vi "Trim All Quots String _APTLib.vi"(7 "Case (NoChange)":T1, 10 "location (both)":T2 items=["both", "start of string", "end of string"], 11 "String In":string) -> (3 "String Out":string)   [LabVIEW 2019]
doc: "This VI is Developed by Anish Prabu.\n\nCopyright © 2006, email:anishprabu243@yahoo.co.in.\nAll rights reserved."
uses:
  <userlib>/APTLib.lnk/String/_Trim String _APTLib.llb/WS _APTLib.ctl
  <userlib>/APTLib.lnk/String/_Trim String _APTLib.llb/Change Case Selector _APTLib.ctl
  <userlib>/APTLib.lnk/String/_Trim String _APTLib.llb/Trim WS (String) _APTLib.vi
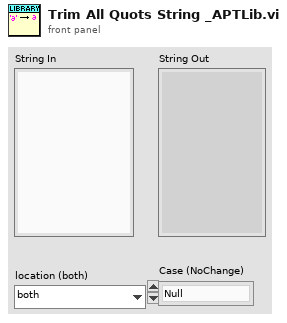
[diagram p1: front panel]
types:
  T1 = typedef "Change Case Selector _APTLib.ctl" = enum16{"Null", "CAPS", "small", "Title", "Sentence"}
  T2 = typedef "WS _APTLib.ctl" = u16
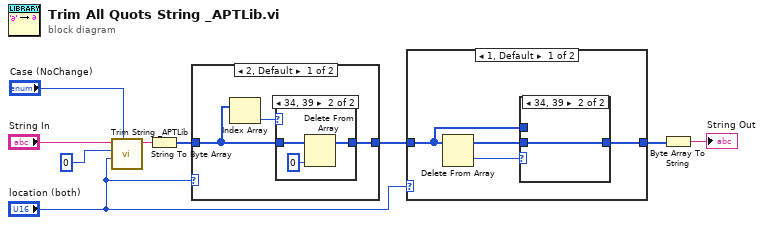
[diagram p0: block diagram]
diagram:
  n1 = call-poly <userlib>:"Trim String _APTLib.vi"("Case (NoChange)"="Case (NoChange)", "location (both)"="location (both)", "length(0)"=0, "String In"="String In") -> ("String Out"=w3:string)  [unwired: 7 in]
  n2 = String To Byte Array(string=w3) -> (unsigned byte array=w9:u8[])
  n3 = case shown="2, Default" "location (both)" {
    tunnel: w9 -> [w11 w17]
    tunnel: [w12 w17] -> w8
    frame 2, Default {
      n4 = Index Array(array=w11) -> (element=w10:u8)  [unwired: 1 in]
      n5 = case shown="34, 39" w10 {
        tunnel: [w13 w16] -> w12
        tunnel: w11 -> [w13 w15]
        frame 0, Default {
        }
        frame 34, 39 {
          n6 = Delete From Array(array=w15, index=0) -> (array with subset deleted=w16:u8[])  [unwired: 1 in, 1 out]
        }
      }
    }
    frame 1 {
    }
  }
  n7 = case shown="1, Default" "location (both)" {
    tunnel: w8 -> [w18 w24]
    tunnel: [w19 w24] -> w7
    frame 1, Default {
      n8 = Delete From Array(array=w18) -> (deleted portion=w21:u8, array with subset deleted=w20:u8[])  [unwired: 2 in]
      n9 = case shown="34, 39" w21 {
        tunnel: w20 -> [_ w23]
        tunnel: [w22 w23] -> w19
        tunnel: w18 -> [w22 _]
        frame 0, Default {
        }
        frame 34, 39 {
        }
      }
    }
    frame 2 {
    }
  }
  n10 = Byte Array To String(unsigned byte array=w7) -> (string=→"String Out":string)
